vi "SpedUpAutonomous.vi"   [LabVIEW 2014]
uses:
  Robot Global Data.vi
  <vilib>/Rock Robotics/WPI/Solenoid/Deprecated/WPI_SolenoidSetBool.vi
types:
  T1 = typedef "WPI_SolenoidDevRef.ctl" = cluster{"DevStatus":errorcluster, "Pneumatics Control Module":u8, "Forward Solenoid Channel":T2, "Reverse Solenoid Channel":T2}
  T2 = typedef "WPI_SolenoidChannel.ctl" = enum8{"Solenoid 0", "Solenoid 1", "Solenoid 2", "Solenoid 3", "Solenoid 4", "Solenoid 5", "Solenoid 6", "Solenoid 7", "Invalid"}
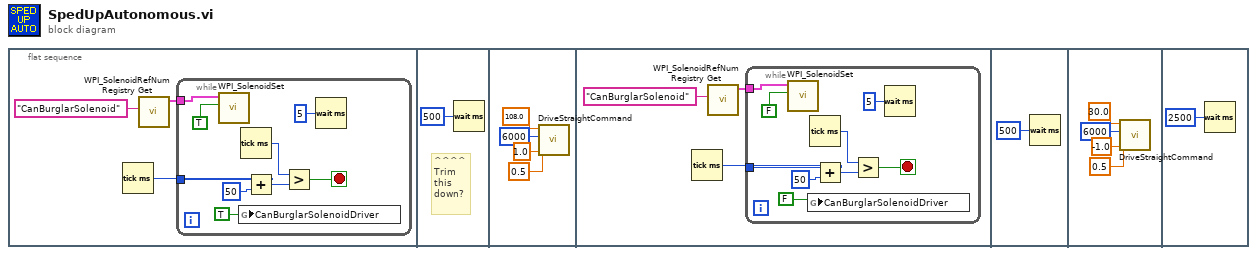
[diagram p0: block diagram]
diagram:
  n1 = flat-sequence {
    frame #0 {
      n2 = Tick Count (ms)() -> (millisecond timer value=w3:u32)
      n3 = call <vilib>:"WPI_SolenoidRefNum Registry Get.vi"("refnum name"="CanBurglarSolenoid") -> ("SolenoidDevRef"=w1:T1)  [unwired: 9 in, 1 out]
      n4 = while {
        tunnel: w3 -> [w12]
        tunnel: w1 -> [w6]
        stop <- w8 stop-if-true
        n5 = call-poly <vilib>:"WPI_SolenoidSet.vi"("Value"=TRUE ("CanBurglarSolenoidDriver"), "SolenoidDevRef"=w6) -> ()  [unwired: 8 in, 2 out]
        n6 = global write "Robot Global Data.vi" "CanBurglarSolenoidDriver"(TRUE ("CanBurglarSolenoidDriver")) -> ()
        n7 = Tick Count (ms)() -> (millisecond timer value=w10:u32)
        n8 = Add(x=w12, y=u32 50) -> (x+y=w9:u32)
        n9 = Greater?(x=w10, y=w9) -> (0:w8:bool)
        n10 = Wait (ms)(milliseconds to wait=u32 5) -> ()  [unwired: 1 out]
      }
    }
    frame #1 {
      # "^^^^\nTrim\nthis\ndown?"
      n11 = Wait (ms)(milliseconds to wait=u32 500) -> ()  [unwired: 1 out]
    }
    frame #2 {
      n12 = call "DriveStraightCommand.vi"("speed"=0.5, "Fwd Bwd"=1.0, "Delay ms"=u32 6000, "distance"=108.0) -> ()  [unwired: 8 in]
    }
    frame #3 {
      n13 = Tick Count (ms)() -> (millisecond timer value=w20:u32)
      n14 = call <vilib>:"WPI_SolenoidRefNum Registry Get.vi"("refnum name"="CanBurglarSolenoid") -> ("SolenoidDevRef"=w18:T1)  [unwired: 9 in, 1 out]
      n15 = while {
        tunnel: w20 -> [w29]
        tunnel: w18 -> [w23]
        stop <- w25 stop-if-true
        n16 = call-poly <vilib>:"WPI_SolenoidSet.vi"("Value"=FALSE ("CanBurglarSolenoidDriver"), "SolenoidDevRef"=w23) -> ()  [unwired: 8 in, 2 out]
        n17 = global write "Robot Global Data.vi" "CanBurglarSolenoidDriver"(FALSE ("CanBurglarSolenoidDriver")) -> ()
        n18 = Tick Count (ms)() -> (millisecond timer value=w27:u32)
        n19 = Add(x=w29, y=u32 50) -> (x+y=w26:u32)
        n20 = Greater?(x=w27, y=w26) -> (0:w25:bool)
        n21 = Wait (ms)(milliseconds to wait=u32 5) -> ()  [unwired: 1 out]
      }
    }
    frame #4 {
      n22 = Wait (ms)(milliseconds to wait=u32 500) -> ()  [unwired: 1 out]
    }
    frame #5 {
      n23 = call "DriveStraightCommand.vi"("speed"=0.5, "Fwd Bwd"=-1.0, "Delay ms"=u32 6000, "distance"=30.0) -> ()  [unwired: 8 in]
    }
    frame #6 {
      n24 = Wait (ms)(milliseconds to wait=u32 2500) -> ()  [unwired: 1 out]
    }
  }
